vi "init_set_length_waveform.vi"(11 "waveform":waveform(dbl)) -> (3 "output waveform":waveform(dbl))   [LabVIEW 2017]
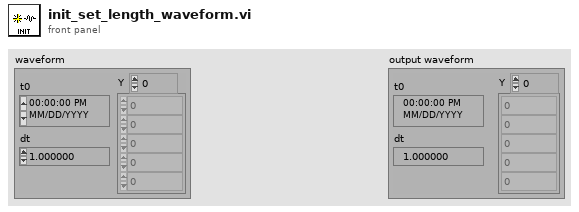
[diagram p1: front panel]
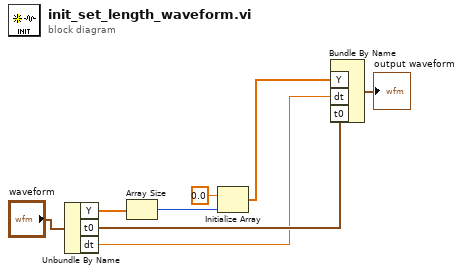
[diagram p0: block diagram]
diagram:
  n1 = Unbundle By Name("waveform") -> ("Y"=w8:dbl[], "t0"=w4:timestamp, "dt"=w1:dbl)
  n2 = Array Size(array=w8) -> (size(s)=w7:i32)
  n3 = Initialize Array(0.0 ("element"), w7) -> (w5:dbl[])
  n4 = Bundle By Name("Y"=w5, "dt"=w1, "t0"=w4) -> (→"output waveform":waveform(dbl))  [unwired: 1 in]
